vi "Read Dual Fan Actor.vi"(11 "仿真冷却器":refnum<class "Simulated Evaporative Cooler.lvclass">) -> (2 "双风扇":refnum<class "Dual Fan.lvclass">)   [LabVIEW 2015, in "Simulated Evaporative Cooler.lvclass"]
uses:
  Simulated Evaporative Cooler.lvclass
  Dual Fan/Dual Fan/Dual Fan.lvclass
  Simulated Dual Fan/Simulated Dual Fan.lvclass
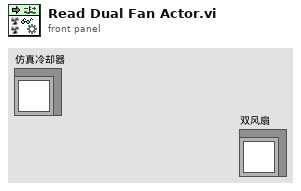
[diagram p1: front panel]
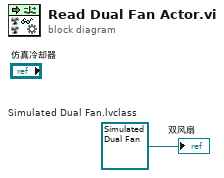
[diagram p0: block diagram]
diagram:
  w1 = refnum<class "Simulated Dual Fan.lvclass"> refnum  # Simulated Dual Fan.lvclass
  "双风扇" <- w1
